vi "TCP Read.vi"(8 "error in (no error)":errorcluster caption="错误输入（无错误）", 11 "连接ID":refnum<k5>) -> (0 "error out":errorcluster caption="错误输出", 2 "数据输出":string, 3 "连接ID输出":refnum<k5>)   [LabVIEW 2017]
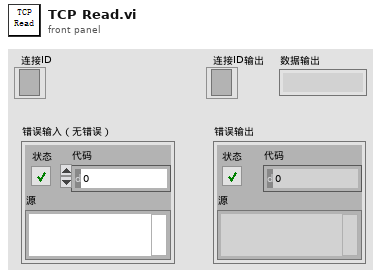
[diagram p1: front panel]
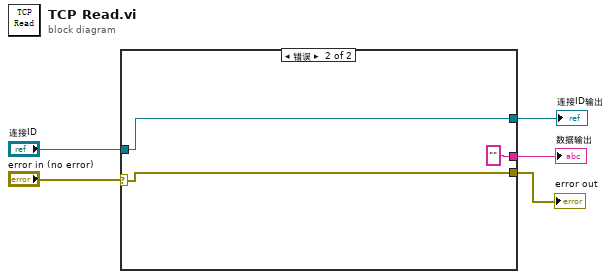
[diagram p0: block diagram]
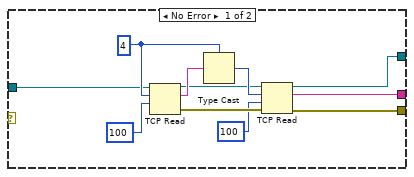
[diagram p2: hidden frame]
diagram:
  n1 = case shown="错误" "error in (no error)" {
    selector: "error in (no error)" -> [_ w19]
    tunnel: [w9 w19] -> w4
    tunnel: "连接ID" -> [w8 w18]
    tunnel: [w7 "" ("data out")] -> w2
    tunnel: [w6 w18] -> w1
    frame No Error {
      w12 = 4
      n2 = TCP Read(connection ID=w8, bytes to read=w12, 9:100 ("超时毫秒(25000)")) -> (connection ID out=w14:refnum<k5>, data out=w16:string, error out=w13:errorcluster)  [unwired: 2 in]
      n3 = Type Cast(type=w12, x=w16) -> (*(type *) &x=w15:i32)
      n4 = TCP Read(connection ID=w14, bytes to read=w15, error in (no error)=w13, 9:100 ("超时毫秒(25000)")) -> (connection ID out=w6:refnum<k5>, data out=w7:string, error out=w9:errorcluster)  [unwired: 1 in]
    }
    frame Error {
    }
  }
  "error out" <- w4
  "连接ID输出" <- w1
  "数据输出" <- w2
